vi "TL behavior S-Wall_D.vi"(1 "Behavior\nVelocity":dbl, 2 "Activate?":bool=TRUE, 3 "Sensor":T1) -> (0 "S-Wall Array":dbl[](array[numeric]))   [LabVIEW 2014]
uses:
  sensorsSTD.ctl
  <vilib>/addons/control/pid/pid.llb/PID (DBL).vi
  <vilib>/addons/control/pid/NI_PID_pid.lvlib
panel:
  out "Sensor C":string
  in  "setpoint 0deg":dbl=15.0 format="%#_13g"
  out "steer 0":dbl format="%.2f"
  in  "setpoint 90deg":dbl=20.0 format="%#_13g"
  out "steer 90":dbl format="%.2f"
  out "Sensor B":string
  out "Sensor A":string
  in  "setpoint 45deg":dbl=35.0 format="%#_13g"
  out "steer 45":dbl format="%.2f"
  out "Waveform Graph":cluster{dbl, dbl, dbl[]}(graph)
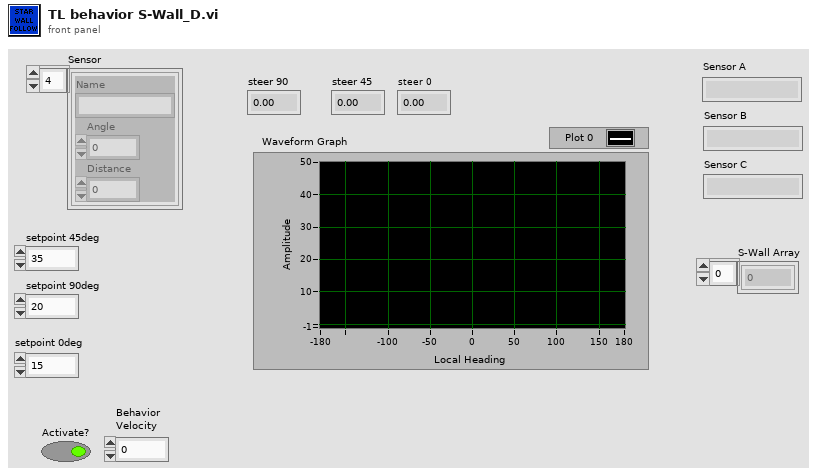
[diagram p1: front panel]
types:
  T1 = typedef "sensorsSTD.ctl" = cluster{"Name":string, "Angle":dbl, "Distance":dbl}[]
  T2 = cluster{"proportional gain (Kc)":dbl, "integral time (Ti, min)":dbl, "derivative time (Td, min)":dbl}
  T3 = cluster{"Name":string, "Angle":dbl, "Distance":dbl}
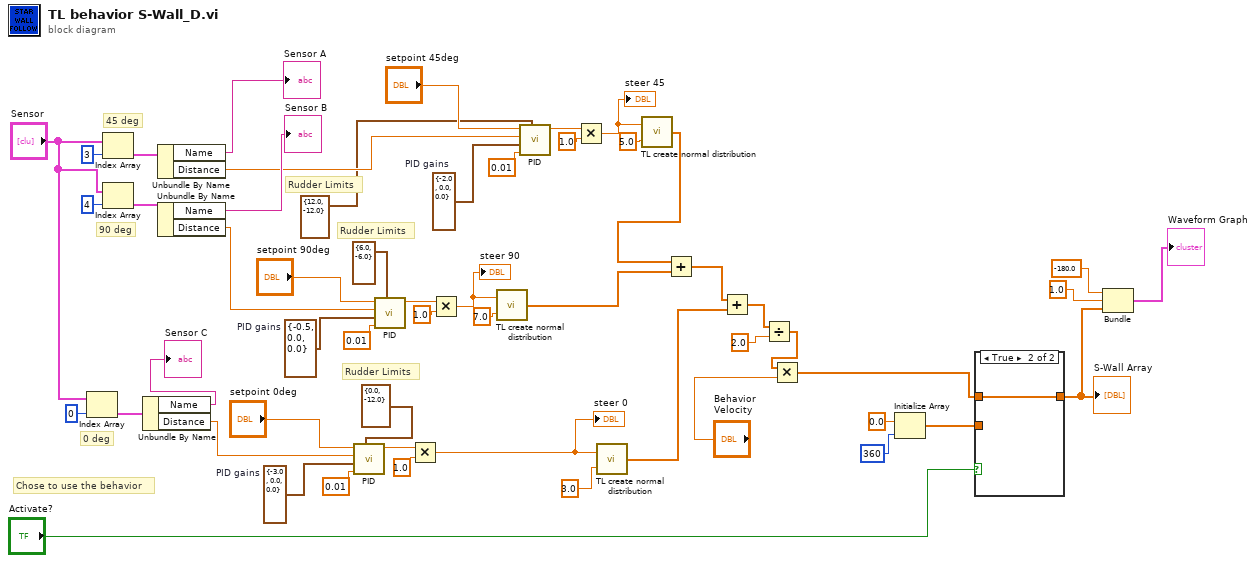
[diagram p0: block diagram]
diagram:
  w14 = T2 {"proportional gain (Kc)"=-3.0, "integral time (Ti, min)"=0.0, "derivative time (Td, min)"=0.0}  # PID gains
  w31 = T2 {"proportional gain (Kc)"=-0.5, "integral time (Ti, min)"=0.0, "derivative time (Td, min)"=0.0}  # PID gains
  w39 = T2 {"proportional gain (Kc)"=-2.0, "integral time (Ti, min)"=0.0, "derivative time (Td, min)"=0.0}  # PID gains
  # "Rudder Limits"
  # "Rudder Limits"
  # "0 deg"
  # "90 deg"
  # "45 deg"
  # "Rudder Limits"
  # "Chose to use the behavior"
  n1 = Index Array(array="Sensor", index=0) -> (element=w18:T3)
  n2 = Index Array(array="Sensor", index=3) -> (element=w53:T3)
  n3 = Index Array(array="Sensor", index=4) -> (element=w43:T3)
  n4 = Unbundle By Name(w18) -> ("Name"=→"Sensor C":string, "Distance"=w9:dbl)
  n5 = Unbundle By Name(w53) -> ("Name"=→"Sensor A":string, "Distance"=w27:dbl)
  n6 = Unbundle By Name(w43) -> ("Name"=→"Sensor B":string, "Distance"=w28:dbl)
  n7 = call-poly <vilib>:"PID.vi"("output range"=cluster{"output high":dbl, "output low":dbl} {"output high"=0.0, "output low"=-12.0}, "dt (s)"=0.01, "PID gains"=w14, "process variable"=w9, "setpoint"="setpoint 0deg") -> ("output"=w17:dbl)  [unwired: 5 in, 1 out]
  n8 = call-poly <vilib>:"PID.vi"("output range"=cluster{"output high":dbl, "output low":dbl} {"output high"=6.0, "output low"=-6.0}, "dt (s)"=0.01, "PID gains"=w31, "process variable"=w28, "setpoint"="setpoint 90deg") -> ("output"=w34:dbl)  [unwired: 5 in, 1 out]
  n9 = Multiply(x=w17, y=1.0) -> (x*y=w5:dbl)
  "steer 0" <- w5
  n10 = Multiply(x=w34, y=1.0) -> (x*y=w30:dbl)
  "steer 90" <- w30
  n11 = call "TL create normal distribution.vi"("std (Normal)"=7.0, "mean"=w30) -> ("ACT array"=w25:dbl[])
  n12 = call-poly <vilib>:"PID.vi"("output range"=cluster{"output high":dbl, "output low":dbl} {"output high"=12.0, "output low"=-12.0}, "dt (s)"=0.01, "PID gains"=w39, "process variable"=w27, "setpoint"="setpoint 45deg") -> ("output"=w42:dbl)  [unwired: 5 in, 1 out]
  n13 = Multiply(x=w42, y=1.0) -> (x*y=w38:dbl)
  "steer 45" <- w38
  n14 = call "TL create normal distribution.vi"("std (Normal)"=3.0, "mean"=w5) -> ("ACT array"=w10:dbl[])
  n15 = call "TL create normal distribution.vi"("std (Normal)"=5.0, "mean"=w38) -> ("ACT array"=w26:dbl[])
  n16 = Add(x=w26, y=w25) -> (x+y=w11:dbl[])
  n17 = Add(x=w11, y=w10) -> (x+y=w4:dbl[])
  n18 = Divide(x=w4, y=2.0) -> (x/y=w3:dbl[])
  n19 = Multiply(x=w3, y="Behavior\nVelocity") -> (x*y=w23:dbl[])
  n20 = Initialize Array(0.0 ("element"), 360 ("dimension size")) -> (w46:dbl[])
  n21 = case shown="True" "Activate?" {
    tunnel: w46 -> [w55 _]
    tunnel: w23 -> [_ w56]
    tunnel: [w55 w56] -> w45
    frame False {
    }
    frame True {
    }
  }
  "S-Wall Array" <- w45
  n22 = Bundle(-180.0, 1.0, w45) -> (→"Waveform Graph":cluster{dbl, dbl, dbl[]})  [unwired: 1 in]
